vi "Send Current.vi"(8 "error in":errorcluster, 11 "69X_79X in":refnum<class "79XRP.lvclass">) -> (0 "error out":errorcluster, 3 "69X_79X out":refnum<class "79XRP.lvclass">)   [LabVIEW 2019, in "79XRP.lvlib" / "79XRP.lvclass"]
uses:
  Library/79XRP.lvclass
  C:/Users/Public/Documents/Development/builds/Instruments/PowerSupply.lvlibp/Library/PowerSupply.lvclass
  Accessors/Read Local Resource.vi
  Accessors/Write Local Resource.vi
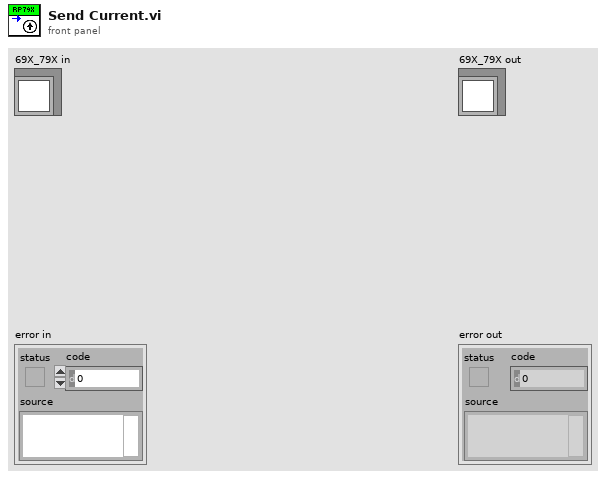
[diagram p1: front panel]
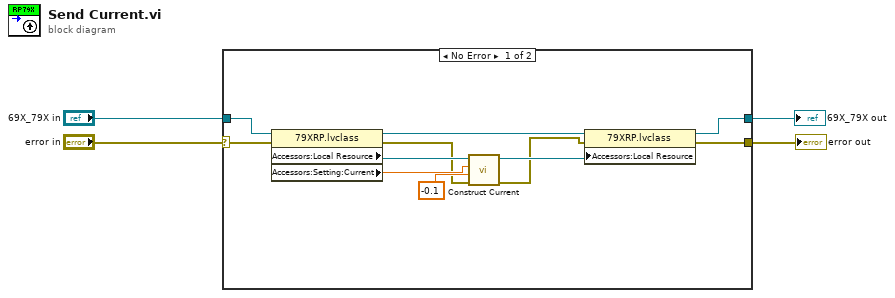
[diagram p0: block diagram]
diagram:
  n1 = case shown="No Error" "error in" {
    selector: "error in" -> [w14 w16]
    tunnel: "69X_79X in" -> [w15 w17]
    tunnel: [w11 w17] -> w4
    tunnel: [w12 w16] -> w3
    frame No Error {
      n2 = property class="79XRP.lvclass"(reference=w15, error in=w14) -> (reference out=w13:refnum<class "79XRP.lvclass">, error out=w6:errorcluster, "Accessors:Local Resource"=w10:refnum<visa-resource-name>, "Accessors:Setting:Current"=w8:dbl)
      n3 = call "Construct Current.vi"("error in (no error)"=w6, "Negative Current Limit"=-0.1, "Positive Current Limit"=w8, "VISA resource name"=w10) -> ("error out"=w5:errorcluster, "VISA resource name out"=w9:refnum<visa-resource-name>)  [unwired: 6 in]
      n4 = property class="79XRP.lvclass"(reference=w13, error in=w5, "Accessors:Local Resource"=w9) -> (reference out=w11:refnum<class "79XRP.lvclass">, error out=w12:errorcluster)
    }
    frame Error {
    }
  }
  "error out" <- w3
  "69X_79X out" <- w4
